vi "sendOnExchange.vi"(0 "RabbitMQ Session In":T1, 5 "Exchange Name in":string, 7 "Routing Key in":string, 9 "Message In":string, 11 "error in (no error)":errorcluster) -> (4 "RabbitMQ Session Out":T1, 6 "Exchange Name out":string, 8 "Routing Key out":string, 10 "Message out":string, 15 "error out":errorcluster)   [LabVIEW 2019, in "rabbitmq.lvlib"]
uses:
  rabbitmq.lvlib
  session.ctl
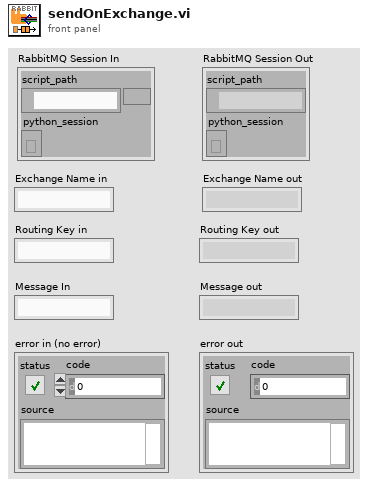
[diagram p1: front panel]
types:
  T1 = typedef "rabbitmq.lvlib/session.ctl" = cluster{"script_path":path, "python_session":refnum<k35>}
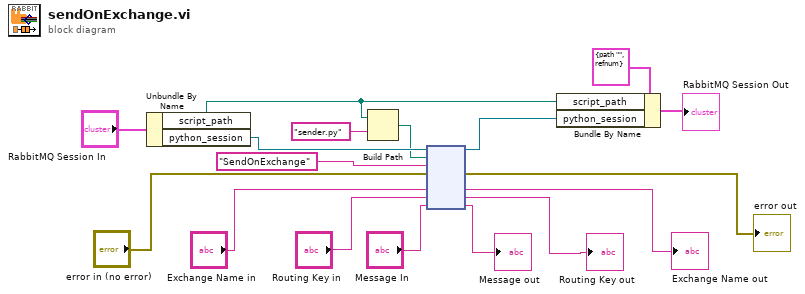
[diagram p0: block diagram]
diagram:
  n1 = Unbundle By Name("RabbitMQ Session In") -> ("script_path"=w8:path, "python_session"=w12:refnum<k35>)
  n2 = Build Path(base path=w8, name or relative path="sender.py") -> (appended path=w7:path)
  n3 = node(w12, w7, "SendOnExchange" ("function name"), "error in (no error)", "Exchange Name in", "Routing Key in", "Message In") -> (w17:refnum<k35>, →"error out":errorcluster, →"Exchange Name out":string, →"Routing Key out":string, →"Message out":string)  [unwired: 2 in, 2 out]
  n4 = Bundle By Name(cluster=T1 {"script_path"=path "", "python_session"=refnum}, "script_path"=w8, "python_session"=w17) -> (→"RabbitMQ Session Out":T1)
